vi "0 OCU.vi"(9 "Overview Image Ref In":T9, 10 "Map Name":T3="LPB Pool", 11 "Location of THINK":T13="127.0.0.1") -> ()   [LabVIEW 2011]
doc: "This is the current implementation of the operator control unit (OCU) for small RC boat controlled by a host computer. The following features are currently implemented:\n- override control of the rudden angle and sail value by control interface or using keys\n- ability to add missions before and during a run, by clicking and by using GPS location of the boat or an auxiliary GPS attached to the OCU computer\n- modification of tuning values used on the boat\n- indicators for all relevant system status information\n\nAuthors: Jared Kirschner, Jason Curtis"
uses:
  2-Think/2 Typedefs/setpoints to boat.ctl
  2-Think/2 Typedefs/sail setpt.ctl
  2-Think/2 Typedefs/rudder angle.ctl
  2-Think/2 Typedefs/Velocity.ctl
  2-Think/2 Typedefs/apparent wind direction.ctl
  2-Think/2 Typedefs/apparent wind speed.ctl
  2-Think/2 Typedefs/apparent wind.ctl
  2-Think/2 Typedefs/heading.ctl
  2-Think/2 Typedefs/UTM Location.ctl
  2-Think/2 Typedefs/Which Boat.ctl
  2-Think/2 Typedefs/generalized sensor status.ctl
  2-Think/2 Typedefs/indicator LED.ctl
  0x2-OCU-Think Comm/0x2 Typedefs/Current Waypoint.ctl
  2-Think/2 Typedefs/robot velocity.ctl
  0x2-OCU-Think Comm/0x2 Typedefs/manual override.ctl
  0 Typedefs/Location of Think.ctl
  0 Typedefs/Sail Position.ctl
  0 Typedefs/Rudder Position.ctl
  0 Typedefs/Apparent Wind Point of Sail.ctl
  0x2-OCU-Think Comm/0x2 Typedefs/ocuWaypoint.ctl
  0x2-OCU-Think Comm/0x2 Typedefs/Waypoints List.ctl
  2-Think/2 Classes/Waypoint/Waypoint.lvclass
  0 Typedefs/Mission Type Radio Buttons.ctl
  2-Think/2 Typedefs/rate of turn.ctl
  2-Think/2 Typedefs/pitch and roll.ctl
  2-Think/2 Typedefs/PI Constants.ctl
  2-Think/2 Typedefs/Goodness Weightings.ctl
  0 Typedefs/Maps.ctl
  <vilib>/vision/Image Controls.llb/IMAQ Image.ctl
  2-Think/2 Typedefs/Apparent Wind Mode.ctl
  2-Think/2 Classes/Missions/GenericMission/GenericMission.lvclass
  2-Think/2 Typedefs/UTM Circle.ctl
  0x2-OCU-Think Comm/0x2 Typedefs/RIO-OCU update controls.ctl
  2-Think/2 Typedefs/generalized actuator status.ctl
  2-Think/2 Typedefs/absolute wind direction.ctl
  2-Think/2 Typedefs/absolute wind speed.ctl
  2-Think/2 Typedefs/absolute water current vector.ctl
  2-Think/2 Typedefs/Goodness Fns Indicator.ctl
  2-Think/2 Typedefs/eStopCommand.ctl
  0x2-OCU-Think Comm/0x2 Typedefs/ocuMessage.ctl
  0x2-OCU-Think Comm/0x2 Typedefs/ocuCommands.ctl
  0x2-OCU-Think Comm/0x2 Typedefs/Control values.ctl
  0x2-OCU-Think Comm/0x2 Classes/NetworkStreams/Reader/readType.ctl
  2-Think/2 Globals/2 Global.vi
  0x2-OCU-Think Comm/0x2 Classes/NetworkStreams/Reader/NetworkStreamReader.lvclass
  0x2-OCU-Think Comm/0x2 Classes/NetworkStreams/Writer/NetworkStreamWriter.lvclass
  2-Think/2 Classes/Missions/RoundBuoy/RoundBuoy.lvclass
  2-Think/2 Classes/Missions/PassBuoys/PassBuoys.lvclass
  2-Think/2 Classes/Missions/StationKeeping/StationKeeping.lvclass
  2-Think/2 Classes/Missions/Drive/DriveTo.lvclass
panel:
  in  "Enable \nLocal GPS":bool
  out "Sensor Status":T1
  in  "GPS COM port":refnum<visa-resource-name>="COM1"
  in  "Additional inputs":T4(tab)
  in  "Manual Mission Input":enum32{"Drive", "Round", "Pass", "Station"}(tab)
  in  "Waypoint Location":enum32{"0", "1", "2", "3", "4"}(radio)
  in  "Buoy Side":enum32{"Starboard", "Port"}(radio)
  in  "Buoy to Round":enum32{"0", "1", "2", "3", "4"}(radio)
  in  "Starboard Buoy":enum32{"0", "1", "2", "3", "4"}(radio)=enum."1"
  in  "Port Buoy":enum32{"0", "1", "2", "3", "4"}(radio)
  in  "Buoy B":enum32{"0", "1", "2", "3", "4"}(radio)=enum."1"
  in  "Buoy A":enum32{"0", "1", "2", "3", "4"}(radio)
  in  "Add Mission":bool
  in  "Stored Locations Array":T5[](array[typedef])=[{"UTM Zone"=0.0, "Hemisphere"=enum."North", "East"=0.0, "North"=0.0}, {"UTM Zone"=0.0, "Hemisphere"=enum."North", "East"=0.0, "North"=0.0}, {"UTM Zone"=0.0, "Hemisphere"=enum."North", "East"=0.0, "North"=0.0}, {"UTM Zone"=0.0, "Hemisphere"=enum."North", "East"=0.0, "North"=0.0}, {"UTM Zone"=0.0, "Hemisphere"=enum."North", "East"=0.0, "North"=0.0}] {"North" format="%#_10f"; "East" format="%#_8f"}
  in  "Boat to Point 0":bool
  in  "Boat to Point 1":bool
  in  "Boat to Point 2":bool
  in  "Boat to Point 3":bool
  in  "Boat to Point 4":bool
  in  "Local to Point 4":bool
  in  "Local to Point 3":bool
  in  "Local to Point 2":bool
  in  "Local to Point 1":bool
  in  "Local to Point 0":bool
  in  "PI Constants":T6={"Proportional Gain"=1.0, "Integral Time"=0.0, "Derivative Time"=0.0}
  in  "Goodness Weightings":T7={"Target Importance"=0.98, "No Sail Importance"=1.0, "Change Importance"=0.05, "Pure Waypoint \nImportance"=0.0, "Pure Wind \nImportance"=0.0} {"Pure Wind \nImportance" min=0.0 step=0.2; "Pure Waypoint \nImportance" min=0.0 step=0.2; "Change Importance" min=0.0 step=0.2; "No Sail Importance" min=0.0 step=0.2; "Target Importance" min=0.0 step=0.2}
  in  "Update Constants":bool
  in  "No Sail Zone\nTuning Quotient":dbl=0.05 step=0.1
  in  "Heading Change\nWind Adjustment":dbl=0.2 step=0.1
  in  "Waypoint\nTuning Quotient":dbl=80.0 step=0.1
  in  "Apparent Wind Mode":T8 {"Desired Apparent\nWind Direction" step=0.1}
  in  "Runprotection Enabled":bool=TRUE
  in  "Let Sail Out on Windcross":bool
  in  "Shift Goal for currents":bool
  in  "Round Buoy Safety":dbl
  out "Battery Voltage":dbl
  out "Which Boat Am I?":T10
  out "Rudder Position":T11 scale=50.0..-50.0 scale format="%#.2g"
  out "Sail Position":T12
  out "Connected?":bool caption="Connection Status"
  in  "OVERRIDE SAIL?":bool
  in  "OVERRIDE RUDDER?":bool
  in  "Stop":bool
  in  "OCU Tab Control":enum32{"Mission [M]ap", "Detailed [T]elemetry"}(tab)
  in  "Map Mode":enum32{"M[i]ssion Edit", "M[o]nitoring"}(tab)
  in  "Load MDF":bool
  in  "Time(s)":dbl=300.0
  in  "Tolerance":dbl=3.0
  in  "Mission Entry Type":T14
  in  "Mission Def Filepath":path caption="MDF (Mission Definition File) path \n(leave blank for nothing)"
  in  "Reset Missions/Waypts":bool
  in  "Save Waypoints\nand PoI":bool
  out "# of Waypts":i32
  out "Robot Heading":T15 format="%05.1f"
  in  "Plot Colors":T16={"Target"=3381759, "No Sail"=16711680, "Change"=16756736, "Pure Waypt"=35080, "Pure Wind"=16860, "Combined"=16777228}
  out "Goodness Functions":picture
  out "Apparent Wind Direction\nPoint of Sail":T17 scale=0.0..360.0 scale format="%4d"
  out "Runprotection":bool
  in  "Log message":string caption="Log message (type and press enter)"
  in  "Save Image":bool
  out "Mission Map":T9(plugin-control)
  in  "Globals":T18(tab)
  out "Don't Tip?":bool
  out "Wind Sensor Status":T1
  out "Estimated Error":dbl
  out "Robot Heading":T15 format="%05.1f"
  out "Robot UTM Location":T5 {"North" format="%#_10f"; "East" format="%#_8f"}
  out "Robot Velocity":T19
  out "Robot\nRate of Turn":T20 format="%05.1f"
  out "Robot Pitch/Roll":T21 {"Roll" format="%05.1f"; "Pitch" format="%05.1f"}
  out "Absolute Wind":T22 {"East" format="%#_5g"}
  out "Apparent Wind Direction":T23
  out "Apparent Wind Speed":T24
  out "Apparent Wind":T25
  out "Crossing Wind":bool
  out "Setpoints to boat":T26
  out "Sail Position":T27
  out "Rudder Angle":T28
  out "Current Waypoint":T29
  in  "Reset to start":bool
  out "Manual Override":T30
  out "Waypoints Array":T31[](array[typedef]) {"UTM Location"."North" format="%#_10f"; "UTM Location"."East" format="%#_8f"}
  out "Waypoints Object Array":T32
  out "Mission Object Array":refnum<class "GenericMission.lvclass">[](array[class])
  out "Global No Sail Circles":T33[](array[typedef])
  # "Override\nSail: SHIFT"
  # "Override \nRudder: [W]"
  # "Full Out=RIGHT"
  # "Out=UP"
  # "In=DOWN"
  # "Full In=LEFT"
  # "PORT"
  # "STARB"
  # "[A]"
  # "[G]"
  # "Local GPS"
  # "<--[S]"
  # "[D]"
  # "[F]-->"
  # "Note: if THINK\nis on this computer,\nturning on local GPS will do strange things."
  # "HOWTO:\n1. save one or more points by moving GPS sensor to point, and pressing buttons below\n2. choose type of mission from tab control\n3. choose saved point(s) to load into mission. other params come from mission map input above\n4. click \"Add Mission\""
  # "P"
  # "S"
  # "O"
  # "O"
  # "A"
  # "B"
  # "HOWTO:\nchange values here, \nthen hit:"
  # "inputting missions:\nGo To Waypoint: set tolerance, and click on map.\nRound Buoy Port/Starboard: set tolerance, click.\nPass Between Buoys: Click one buoy location\nand drag to the other.\nStation Keeping: click southwest corner, drag to \nsoutheast corner. A square will be generated.\nTime(s) currently unimplemented.\nGlobal No-Sail Zone: click center of zone, drag to edge of\nzone. A circle with appropriate radius will be created."
  # "As Measured"
  # "Path Planning"
  # "From Planning Functions"
  # "(this is not a cluster because subitems\nare generated in parallel code)"
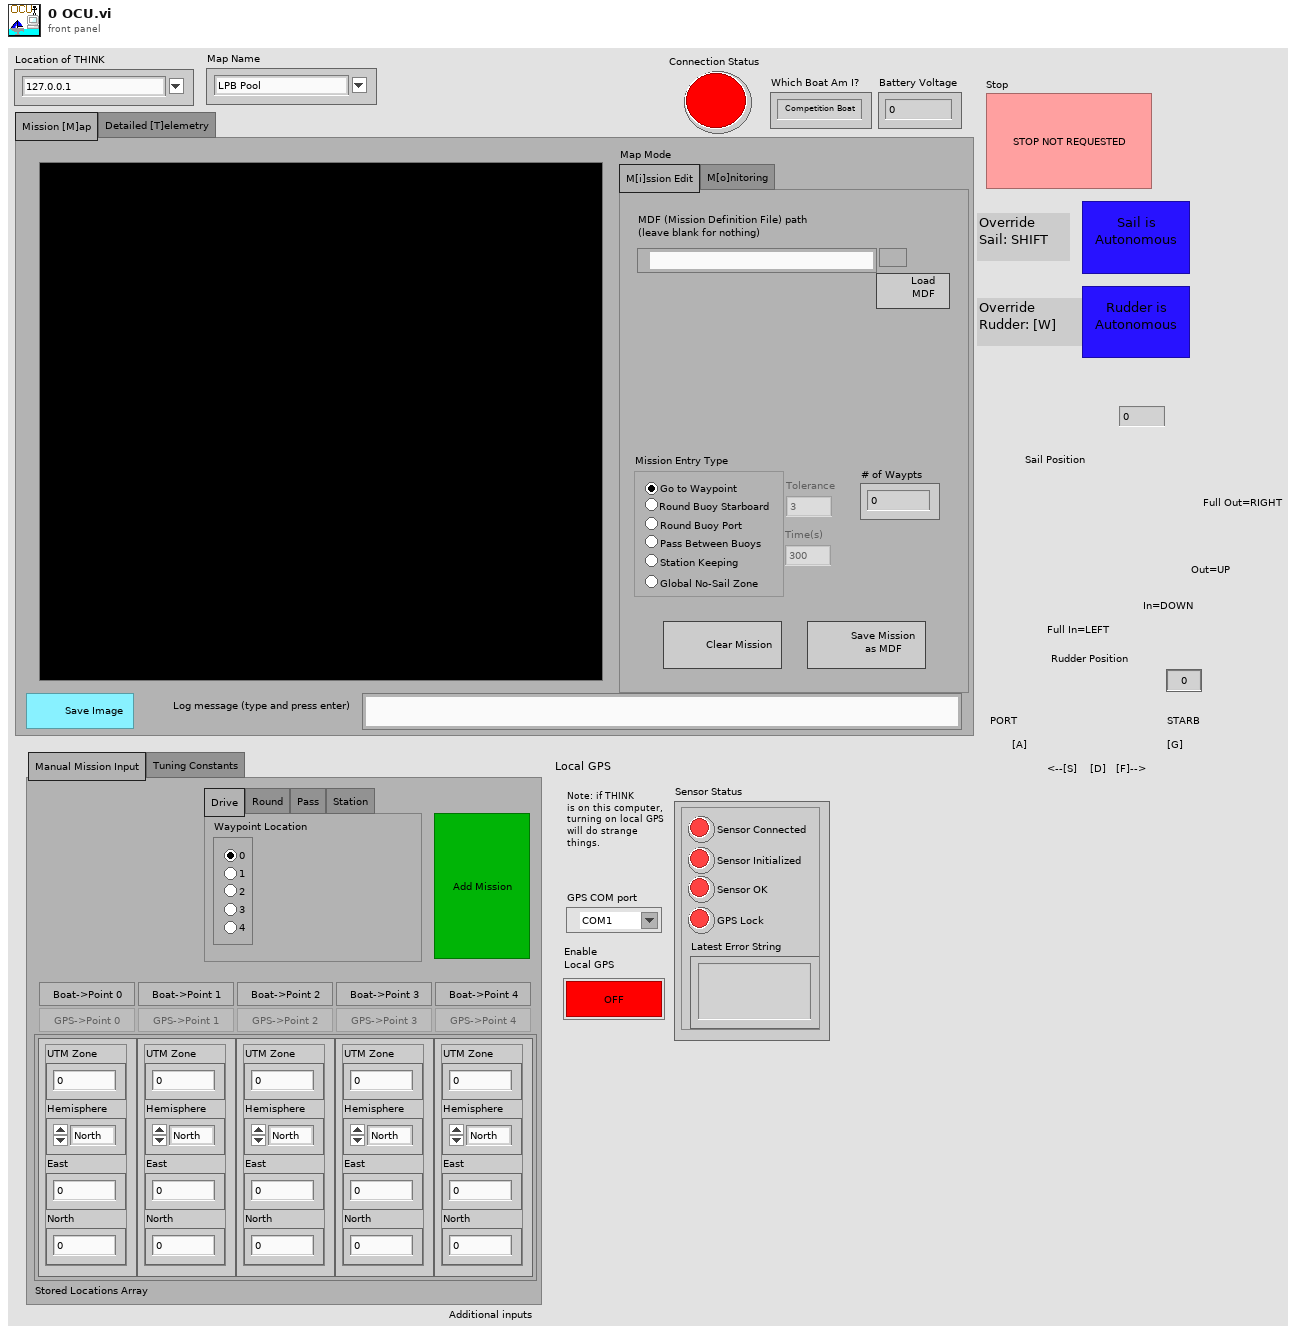
[diagram p1: front panel]
types:
  T1 = typedef "generalized sensor status.ctl" = cluster{"Sensor Connected":T2, "Sensor Initialized":T2, "Sensor OK":T2, "Latest Error String":string, "GPS Lock":T2}
  T2 = typedef "indicator LED.ctl" = bool
  T3 = typedef "Maps.ctl" = string
  T4 = enum32{"Manual Mission Input", "Tuning Constants"}
  T5 = typedef "UTM Location.ctl" = cluster{"UTM Zone":dbl, "Hemisphere":enum16{"North", "South"}, "East":dbl, "North":dbl}
  T6 = typedef "PI Constants.ctl" = cluster{"Proportional Gain":dbl, "Integral Time":dbl, "Derivative Time":dbl}
  T7 = typedef "Goodness Weightings.ctl" = cluster{"Target Importance":dbl, "No Sail Importance":dbl, "Change Importance":dbl, "Pure Waypoint \nImportance":dbl, "Pure Wind \nImportance":dbl}
  T8 = typedef "Apparent Wind Mode.ctl" = cluster{"Desired Apparent\nWind Direction":dbl, "On":bool}
  T9 = typedef "IMAQ Image.ctl" = refnum<image>
  T10 = typedef "Which Boat.ctl" = enum16{"Competition Boat", "Small RC", "Simulation"}
  T11 = typedef "Rudder Position.ctl" = dbl
  T12 = typedef "Sail Position.ctl" = dbl
  T13 = typedef "Location of Think.ctl" = string
  T14 = typedef "Mission Type Radio Buttons.ctl" = enum32{"Go to Waypoint", "Round Buoy Starboard", "Round Buoy Port", "Pass Between Buoys", "Station Keeping", "Global No-Sail Zone"}
  T15 = typedef "heading.ctl" = dbl
  T16 = cluster{"Target":u32, "No Sail":u32, "Change":u32, "Pure Waypt":u32, "Pure Wind":u32, "Combined":u32}
  T17 = typedef "Apparent Wind Point of Sail.ctl" = dbl
  T18 = enum32{"How Am I", "Where Am I", "What's Around Me", "Path Planning"}
  T19 = typedef "robot velocity.ctl" = cluster{"East":dbl, "North":dbl}
  T20 = typedef "rate of turn.ctl" = dbl
  T21 = typedef "pitch and roll.ctl" = cluster{"Pitch":dbl, "Roll":dbl}
  T22 = typedef "Velocity.ctl" = cluster{"East":dbl, "North":dbl}
  T23 = typedef "apparent wind direction.ctl" = dbl
  T24 = typedef "apparent wind speed.ctl" = dbl
  T25 = typedef "apparent wind.ctl" = cluster{"Toward Fore":dbl, "Toward Starboard":dbl}
  T26 = typedef "setpoints to boat.ctl" = cluster{"Sail Position":T27, "Rudder Angle":T28}
  T27 = typedef "sail setpt.ctl" = dbl
  T28 = typedef "rudder angle.ctl" = dbl
  T29 = typedef "Current Waypoint.ctl" = i32
  T30 = typedef "manual override.ctl" = cluster{"Override Active Rudder":bool, "Setpoints":T26, "Override Active Sail":bool}
  T31 = typedef "ocuWaypoint.ctl" = cluster{"Tolerance (m)":dbl, "UTM Location":T5}
  T32 = typedef "Waypoints List.ctl" = refnum<class "Waypoint.lvclass">[]
  T33 = typedef "UTM Circle.ctl" = cluster{"UTM Zone":dbl, "Hemisphere":enum16{"North", "South"}, "East":dbl, "North":dbl, "Radius":dbl}
  T34 = typedef "RIO-OCU update controls.ctl" = cluster{"Sensor Status":T1, "Battery Voltage":dbl, "Rudder Actuator Status":T35, "Sail Actuator Status":T35, "Which Boat Am I?":T10, "Robot Velocity":T19, "Robot UTM Location":T5, "Robot\nHeading ":T15, "Robot\nRate of Turn":T20, "Robot Pitch/Roll":T21, "Apparent Wind":T25, "Apparent Wind\nSpeed":T24, "Apparent Wind\nDirection (º)":T23, "Absolute Wind":T22, "Absolute Wind\nDirection (º)":T36, "Absolute Wind\nSpeed":T37, "Absolute Water Current Vector":T38, "Rudder Angle":T28, "Sail Position":T27, "Manual Override Cluster":T30, "Setpoints to boat":T26, "Current Waypoint":T29, "Think freq.":dbl, "Sense freq.":dbl, "Act freq.":dbl, "E-stop freq.":dbl, "Network \nfreq.":dbl, "Network \nLoop Iterations":i64, "E-Stop":bool, "Serialized Waypoint Array":string, "Serialized Mission Queue Elements":string, "Goodness Functions":T39, "Global No Sail Circles":T33[], "Runprotection":bool, "Optimal Heading":dbl, "Crossing Wind":bool, "Estimated Error":dbl, "Don't Tip?":bool}
  T35 = typedef "generalized actuator status.ctl" = cluster{"Actuator Connected":T2}
  T36 = typedef "absolute wind direction.ctl" = dbl
  T37 = typedef "absolute wind speed.ctl" = dbl
  T38 = typedef "absolute water current vector.ctl" = cluster{"Direction":T23, "Magnitude":T23}
  T39 = typedef "Goodness Fns Indicator.ctl" = cluster{dbl, dbl, dbl[][]}
  T40 = typedef "0-Image Descriptor.ctl" = cluster{"Upper-Left Corner Coordinates":T5, "Meters/Pixel":dbl}
  T41 = typedef "eStopCommand.ctl" = enum16{"Reset E-Stop", "Get E-Stop", "Set E-Stop"}
  T42 = typedef "NetworkStreamReader.lvclass/readType.ctl" = enum16{"Next in buffer", "Most current"}
  T43 = cluster{"Image Ref Out":T9, "Image Descriptor":T40}
  T44 = typedef "ocuMessage.ctl" = cluster{"OCU Command":T45, "Data":variant}
  T45 = typedef "ocuCommands.ctl" = enum16{"Pass", "Send override", "Add waypoint", "Set waypoint number", "Stop", "Add Mission", "Reset Missions/Waypts", "Edit Control Values", "Add Global No-Sail", "Log Message"}
  T46 = typedef "Control values.ctl" = cluster{"Goodness Weightings":T7, "PI Constants":T6, "No Sail Zone\nTuning Quotient":dbl, "Heading Change Wind Adjustment":dbl, "Waypoint Tuning Quotient":dbl, "Apparent Wind Mode":T8, "RP Autonomous":bool, "Let Sail Out on Windcross":bool, "Shift Goal for currents":bool, "Round Buoy Safety":dbl}
  T47 = enum8{"Enabled", "Disabled", "Disabled and Grayed Out"}
  T48 = typedef "eventvkey.ctl" = enum16{"ASCII", "Enter", "Return", "Shift", "Ctrl", "Alt", "Cmd", "Opt", "Caps", "NumLock", "Clear", "Break", "Up", "Down", "Left", "Right", "Insert", "Delete", "Home", "End", "PageUp", "PageDown", "Escape", "Help", "Pause", "ScrollLock", "F1", "F2", "F3", "F4", "F5", "F6", "F7", "F8", "F9", "F10", "F11", "F12", "F13", "F14", "F15", "F16", "F17", "F18", "F19", "F20", "F21", "F22", "F23", "F24", "Play", "VolumeUp", "VolumeDown", "Mute", "Two Byte Char"}
  T49 = cluster{"Global Rectangle":i32[], "Contours":cluster{"Contour Type":u32, "ROI Type":u32, "Points":i32[]}[]}
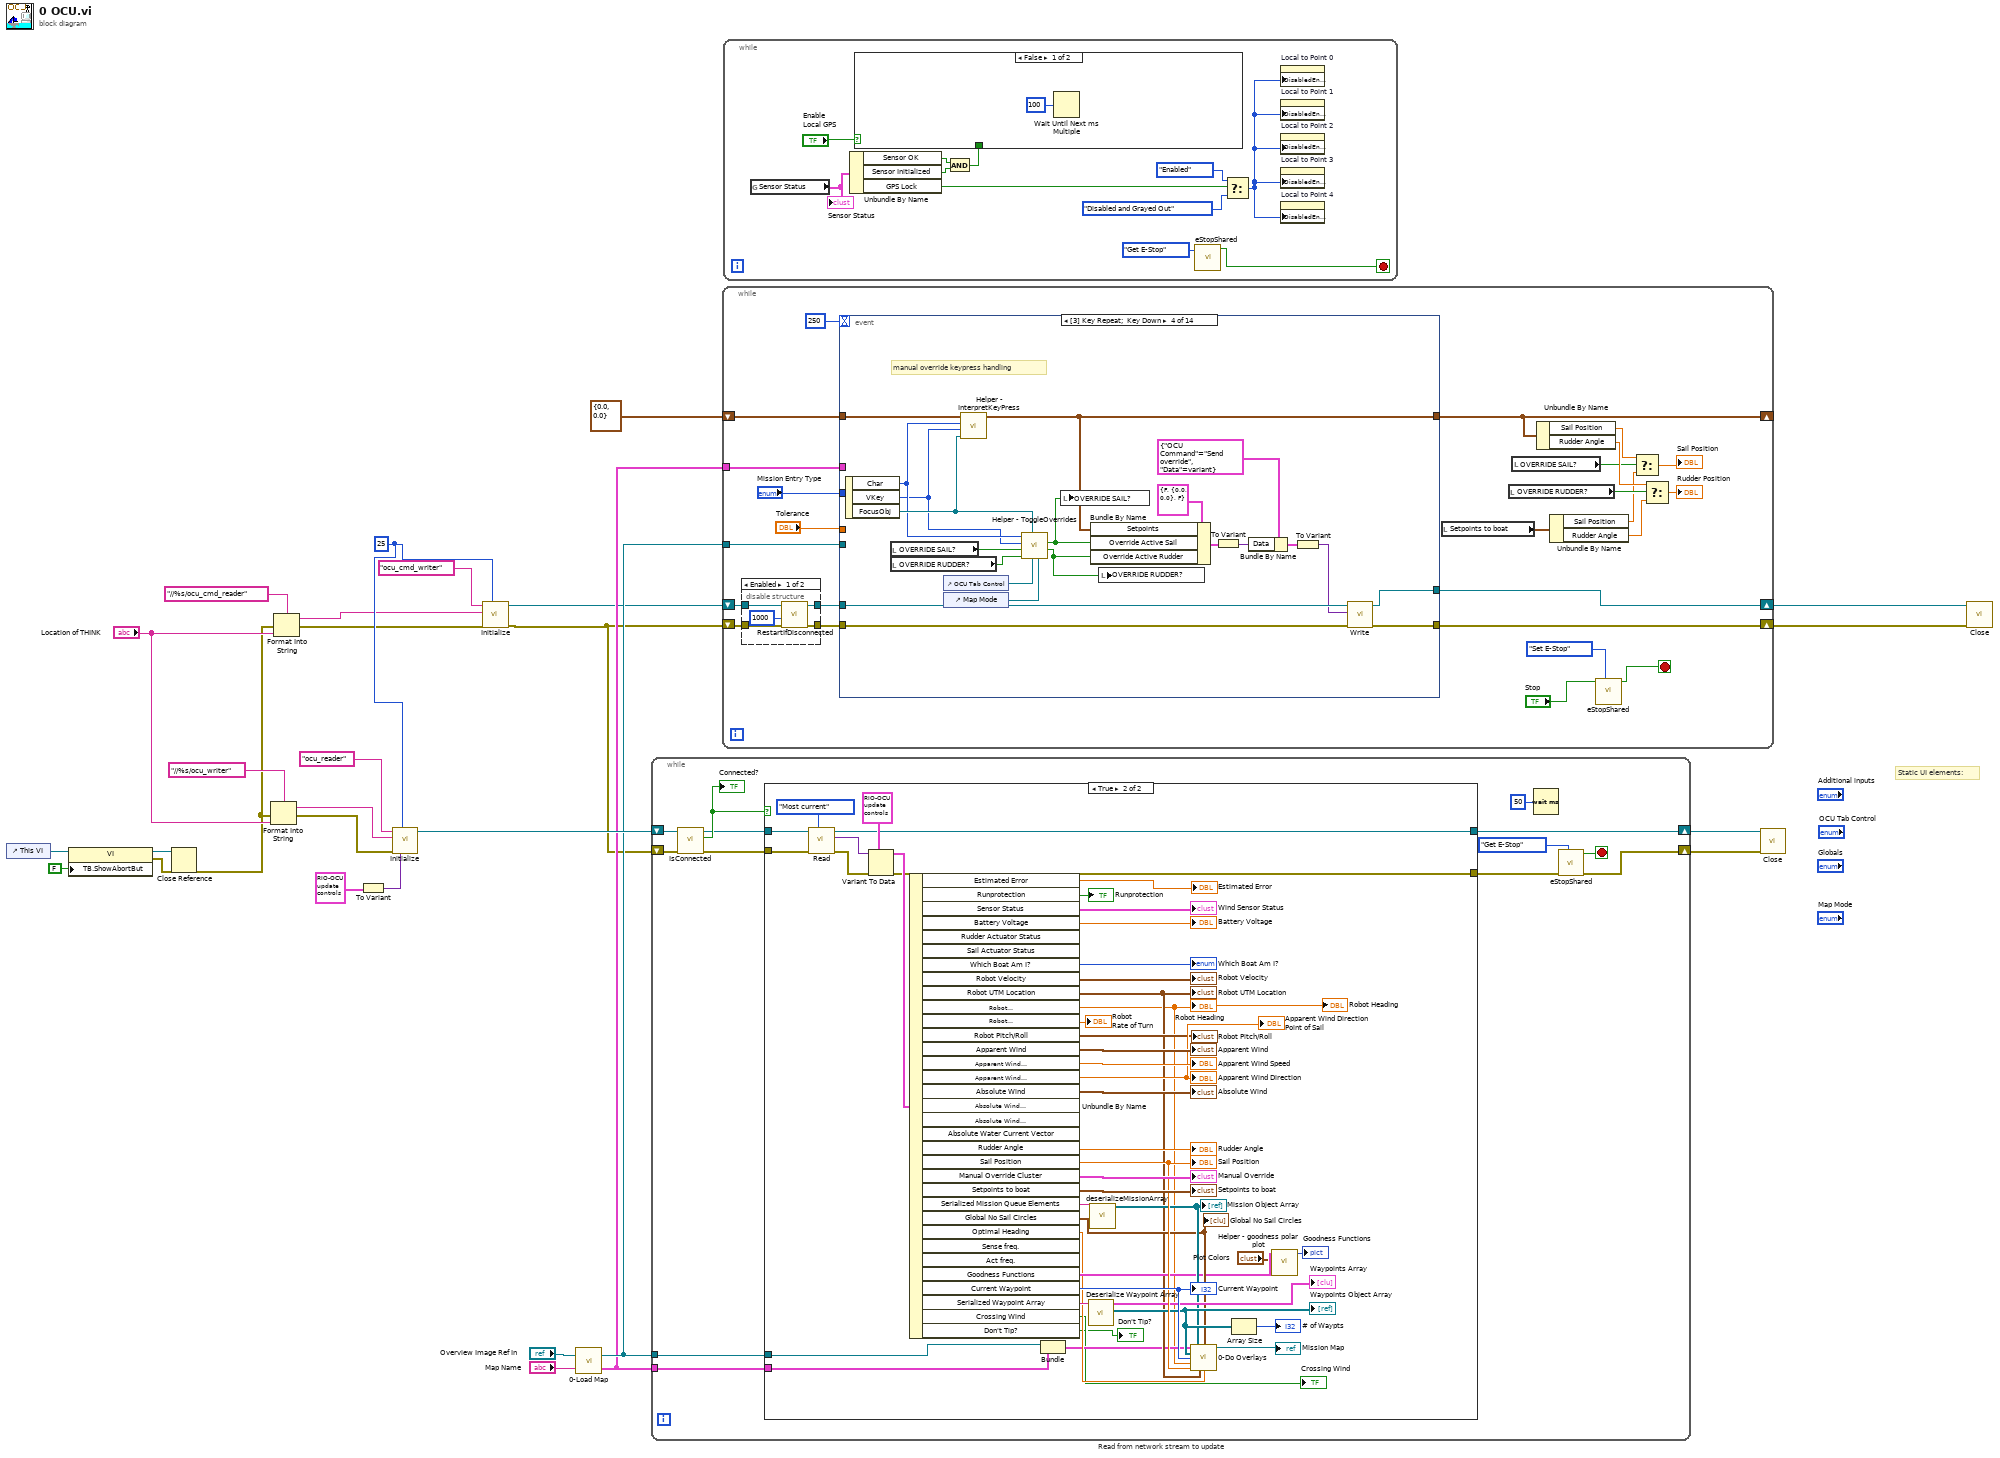
[diagram p0: block diagram]
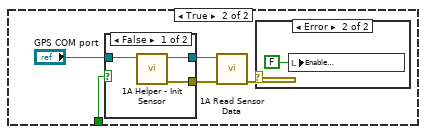
[diagram p2: hidden frame]
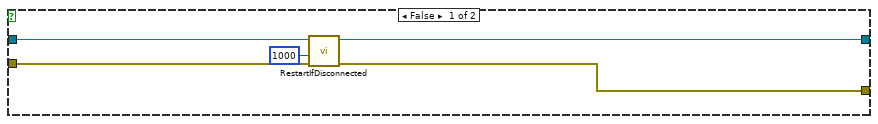
[diagram p5: hidden frame]
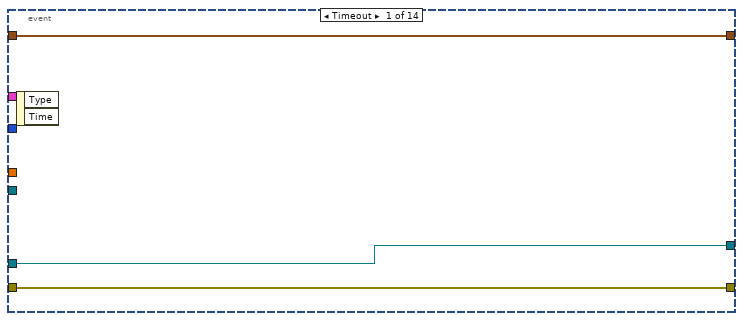
[diagram p7: hidden frame]
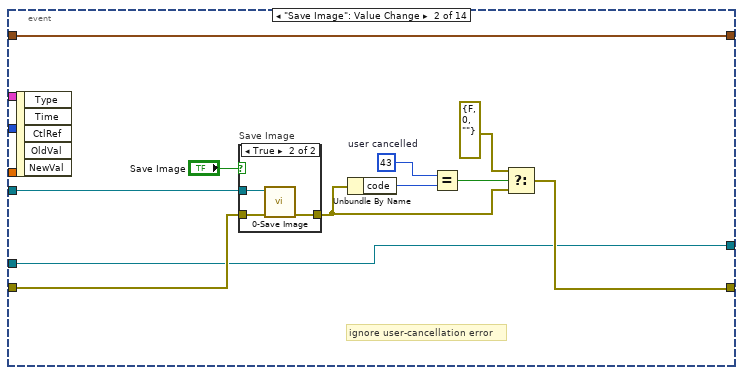
[diagram p8: hidden frame]
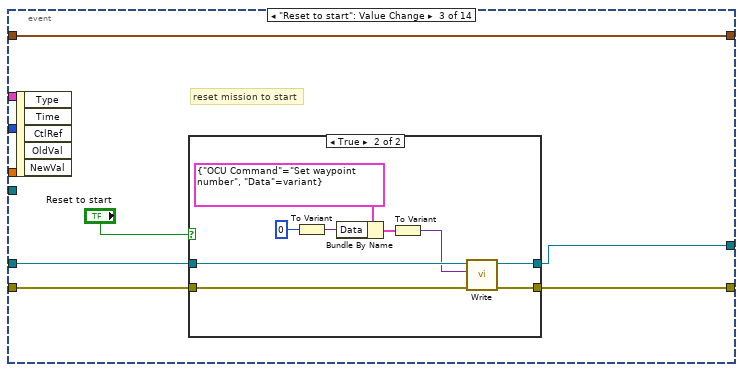
[diagram p10: hidden frame]
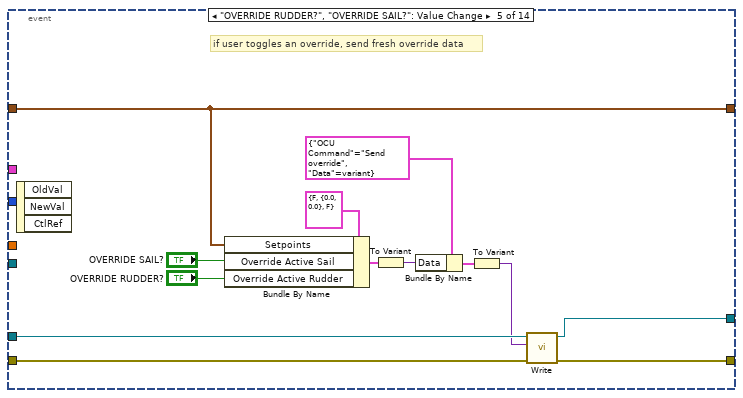
[diagram p12: hidden frame]
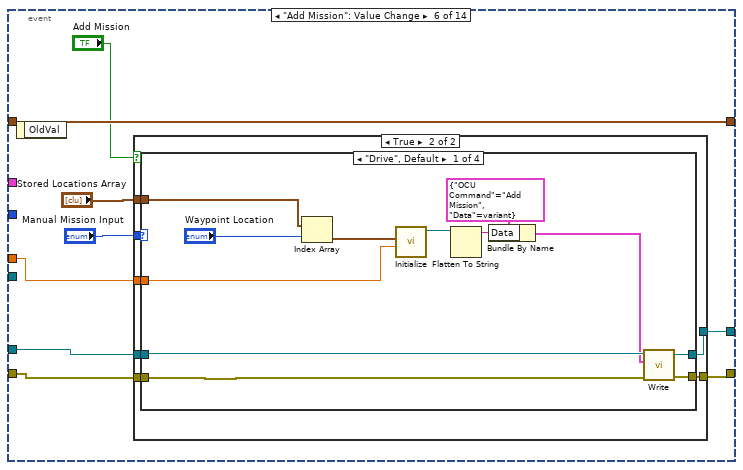
[diagram p13: hidden frame]
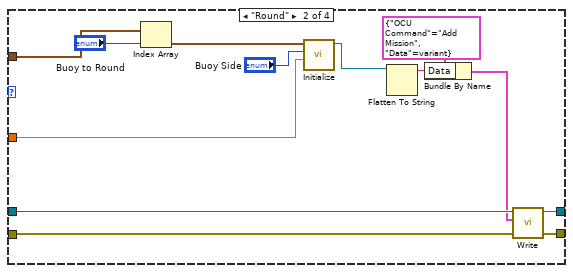
[diagram p15: hidden frame]
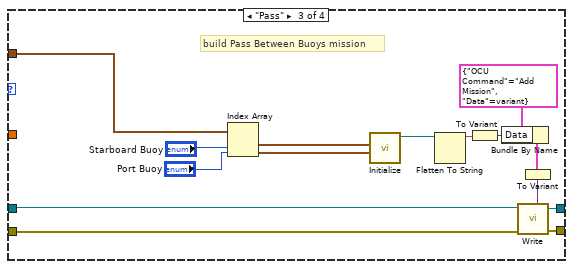
[diagram p16: hidden frame]
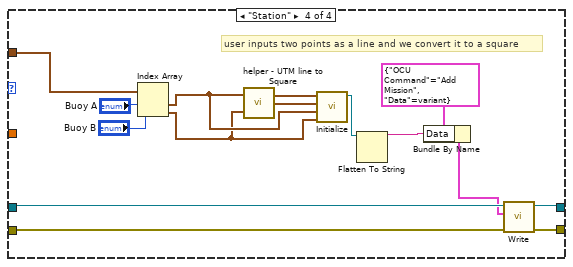
[diagram p17: hidden frame]
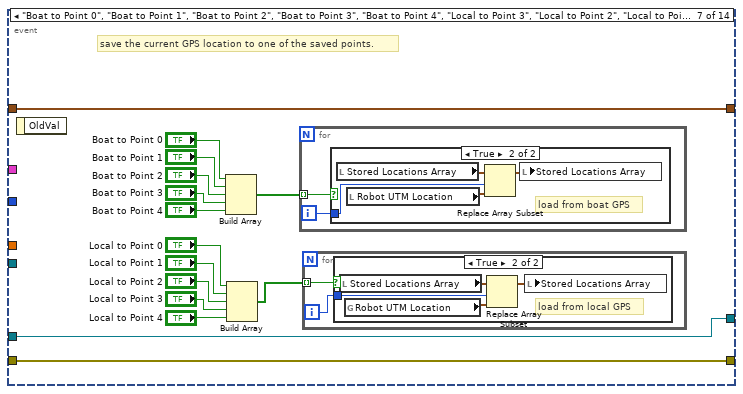
[diagram p18: hidden frame]
diagram:
  w27 = 25 ("writer buffer size")
  # "Static UI elements:"
  n1 = control-ref of="This VI"() -> (w17:refnum<vi>)
  n2 = property class="VI"(reference=w17, "TB.ShowAbortBut"=FALSE ("Tool Bar:Show Abort Button")) -> (reference out=w15:refnum<vi>, error out=w14:errorcluster)  [unwired: 1 in]
  n3 = Close Reference(reference=w15, error in (no error)=w14) -> (error out=w13:errorcluster)
  n4 = Format Into String(format string="//%s/ocu_writer", error in=w13, "Location of THINK") -> (resulting string=w7:string, error out=w11:errorcluster)  [unwired: 1 in]
  n5 = Format Into String(format string="//%s/ocu_cmd_reader", error in=w13, "Location of THINK") -> (resulting string=w5:string, error out=w12:errorcluster)  [unwired: 1 in]
  n6 = To Variant(anything=T34 {"Sensor Status"={"Sensor Connected"=FALSE, "Sensor Initialized"=FALSE, "Sensor OK"=FALSE, "Latest Error String"="", "GPS Lock"=FALSE}, "Battery Voltage"=0.0, "Rudder Actuator Status"={"Actuator Connected"=FALSE}, "Sail Actuator Status"={"Actuator Connected"=FALSE}, "Which Boat Am I?"=enum."Competition Boat", "Robot Velocity"={"East"=0.0, "North"=0.0}, "Robot UTM Location"={"UTM Zone"=0.0, "Hemisphere"=enum."North", "East"=0.0, "North"=0.0}, "Robot\nHeading "=0.0, "Robot\nRate of Turn"=0.0, "Robot Pitch/Roll"={"Pitch"=0.0, "Roll"=0.0}, "Apparent Wind"={"Toward Fore"=0.0, "Toward Starboard"=0.0}, "Apparent Wind\nSpeed"=0.0, "Apparent Wind\nDirection (º)"=0.0, "Absolute Wind"={"East"=0.0, "North"=0.0}, "Absolute Wind\nDirection (º)"=0.0, "Absolute Wind\nSpeed"=0.0, "Absolute Water Current Vector"={"Direction"=0.0, "Magnitude"=0.0}, "Rudder Angle"=0.0, "Sail Position"=0.0, "Manual Override Cluster"={"Override Active Rudder"=FALSE, "Setpoints"={"Sail Position"=0.0, "Rudder Angle"=0.0}, "Override Active Sail"=FALSE}, "Setpoints to boat"={"Sail Position"=0.0, "Rudder Angle"=0.0}, "Current Waypoint"=0, "Think freq."=0.0, "Sense freq."=0.0, "Act freq."=0.0, "E-stop freq."=0.0, "Network \nfreq."=0.0, "Network \nLoop Iterations"=0, "E-Stop"=FALSE, "Serialized Waypoint Array"="", "Serialized Mission Queue Elements"="", "Goodness Functions"={0.0, 0.0, []}, "Global No Sail Circles"=[], "Runprotection"=FALSE, "Optimal Heading"=0.0, "Crossing Wind"=FALSE, "Estimated Error"=0.0, "Don't Tip?"=FALSE} ("RIO->OCU update data")) -> (Variant=w26:variant)
  n7 = call "Initialize.vi"("Default return"=w26, "reader buffer size"=w27, "error in (no error)"=w11, "writer url"=w7, "reader name"="ocu_reader" ("writer name")) -> ("NetworkStreamWriter out"=w28:refnum<class "NetworkStreamReader.lvclass">)  [unwired: 4 in, 2 out]
  n8 = call "Initialize.vi"("writer buffer size"=w27, "error in (no error)"=w12, "reader url"=w5, "writer name"="ocu_cmd_writer") -> ("error out"=w1:errorcluster, "NetworkStreamWriter out"=w2:refnum<class "NetworkStreamWriter.lvclass">)  [unwired: 5 in, 1 out]
  n9 = call "0-Load Map.vi"("Map Name"="Map Name", "Image Ref In"="Overview Image Ref In") -> ("Image Descriptor"=w9:T40, "Image Ref Out"=w23:T9)
  n10 = while "Read from network stream to update" {
    shift-right: [w42] -> w25
    shift-left: w28 -> [w37]
    shift-right: [w35] -> w24
    shift-left: w1 -> [w36]
    tunnel: w23 -> [w39]
    tunnel: w9 -> [w38]
    stop <- w40 stop-if-true
    n11 = call "IsConnected.vi"("error in (no error)"=w36, "NetworkStreamReader in"=w37) -> ("error out"=w31:errorcluster, "Connected?"=w33:bool, "NetworkStreamReader out"=w32:refnum<class "NetworkStreamReader.lvclass">)  [unwired: 7 in]
    "Connected?" <- w33
    n12 = case shown="True" w33 {
      tunnel: [w45 w88] -> w42
      tunnel: w39 -> [_ w65]
      tunnel: w38 -> [_ w64]
      tunnel: w32 -> [w47 w72]
      tunnel: w31 -> [w46 w71]
      tunnel: [w44 w70] -> w30
      frame False {
        n13 = call "RestartIfDisconnected.vi"("error in (no error)"=w46, "connection timeout"=1000, "NetworkStreamReader in"=w47) -> ("error out"=w44:errorcluster, "NetworkStreamReader out"=w45:refnum<class "NetworkStreamReader.lvclass">)  [unwired: 7 in]
      }
      frame True {
        n14 = call "Read.vi"("Read Type"=readType."Most current", "error in (no error)"=w71, "NetworkStreamReader in"=w72) -> ("error out"=w91:errorcluster, "element"=w90:variant, "NetworkStreamReader out"=w88:refnum<class "NetworkStreamReader.lvclass">)  [unwired: 4 in, 2 out]
        n15 = Variant To Data(error in=w91, type=T34 {"Sensor Status"={"Sensor Connected"=FALSE, "Sensor Initialized"=FALSE, "Sensor OK"=FALSE, "Latest Error String"="", "GPS Lock"=FALSE}, "Battery Voltage"=0.0, "Rudder Actuator Status"={"Actuator Connected"=FALSE}, "Sail Actuator Status"={"Actuator Connected"=FALSE}, "Which Boat Am I?"=enum."Competition Boat", "Robot Velocity"={"East"=0.0, "North"=0.0}, "Robot UTM Location"={"UTM Zone"=0.0, "Hemisphere"=enum."North", "East"=0.0, "North"=0.0}, "Robot\nHeading "=0.0, "Robot\nRate of Turn"=0.0, "Robot Pitch/Roll"={"Pitch"=0.0, "Roll"=0.0}, "Apparent Wind"={"Toward Fore"=0.0, "Toward Starboard"=0.0}, "Apparent Wind\nSpeed"=0.0, "Apparent Wind\nDirection (º)"=0.0, "Absolute Wind"={"East"=0.0, "North"=0.0}, "Absolute Wind\nDirection (º)"=0.0, "Absolute Wind\nSpeed"=0.0, "Absolute Water Current Vector"={"Direction"=0.0, "Magnitude"=0.0}, "Rudder Angle"=0.0, "Sail Position"=0.0, "Manual Override Cluster"={"Override Active Rudder"=FALSE, "Setpoints"={"Sail Position"=0.0, "Rudder Angle"=0.0}, "Override Active Sail"=FALSE}, "Setpoints to boat"={"Sail Position"=0.0, "Rudder Angle"=0.0}, "Current Waypoint"=0, "Think freq."=0.0, "Sense freq."=0.0, "Act freq."=0.0, "E-stop freq."=0.0, "Network \nfreq."=0.0, "Network \nLoop Iterations"=0, "E-Stop"=FALSE, "Serialized Waypoint Array"="", "Serialized Mission Queue Elements"="", "Goodness Functions"={0.0, 0.0, []}, "Global No Sail Circles"=[], "Runprotection"=FALSE, "Optimal Heading"=0.0, "Crossing Wind"=FALSE, "Estimated Error"=0.0, "Don't Tip?"=FALSE} ("RIO->OCU update data"), Variant=w90) -> (data=w87:T34, error out=w70:errorcluster)
        n16 = Unbundle By Name(w87) -> ("Estimated Error"=→"Estimated Error":dbl, "Runprotection"=→"Runprotection":bool, "Sensor Status"=→"Wind Sensor Status":T1, "Battery Voltage"=→"Battery Voltage":dbl, "Which Boat Am I?"=→"Which Boat Am I?":T10, "Robot Velocity"=→"Robot Velocity":T19, "Robot UTM Location"=w54:T5, "Robot\nHeading"=w50:T15, "Robot\nRate of Turn"=→"Robot\nRate of Turn":T20, "Robot Pitch/Roll"=→"Robot Pitch/Roll":T21, "Apparent Wind"=→"Apparent Wind":T25, "Apparent Wind\nSpeed"=→"Apparent Wind Speed":T24, "Apparent Wind\nDirection (º)"=→"Apparent Wind Direction" →"Apparent Wind Direction\nPoint of Sail":T23, "Absolute Wind"=→"Absolute Wind":T22, "Rudder Angle"=→"Rudder Angle":T28, "Sail Position"=w73:T27, "Manual Override Cluster"=→"Manual Override":T30, "Setpoints to boat"=→"Setpoints to boat":T26, "Serialized Mission Queue Elements"=w63:string, "Global No Sail Circles"=w59:T33[], "Optimal Heading"=w53:dbl, "Goodness Functions"=w57:T39, "Current Waypoint"=w74:T29, "Serialized Waypoint Array"=w69:string, "Crossing Wind"=→"Crossing Wind":bool, "Don't Tip?"=→"Don't Tip?":bool)  [unwired: 7 out]
        "Robot UTM Location" <- w54
        "Robot Heading" <- w50
        "Sail Position" <- w73
        "Current Waypoint" <- w74
        "Global No Sail Circles" <- w59
        "Robot Heading" <- w50
        n17 = Bundle("Image Ref Out"=w65, "Image Descriptor"=w64) -> (w52:T43)  [unwired: 1 in]
        n18 = call "Deserialize Waypoint Array.vi"("Serialized Waypoint Array"=w69) -> ("Waypoints Object Array"=w67:T32, "Waypoints Array"=→"Waypoints Array":T31[])  [unwired: 9 in]
        "Waypoints Object Array" <- w67
        n19 = call "deserializeMissionArray.vi"("Serialized Mission Array"=w63) -> ("Mission Object Array"=w62:refnum<class "GenericMission.lvclass">[])  [unwired: 9 in, 1 out]
        "Mission Object Array" <- w62
        n20 = call "0-Do Overlays.vi"("Image Reference\nand Descriptor"=w52, "Missions"=w62, "No Sail Circles"=w59, "Waypoints"=w67, "Current Waypoint #"=w74, "Heading"=w50, "Sail Position"=w73, "Robot UTM Location"=w54, "Optimal Heading"=w53) -> ("Image out"=→"Mission Map":T9)  [unwired: 6 in]
        n21 = Array Size(array=w67) -> (size(s)=→"# of Waypts":i32)
        n22 = call "Helper - goodness polar plot.vi"("Plot Colors"="Plot Colors", "Goodness Fns In"=w57) -> ("Goodness Functions Polar Plot"=→"Goodness Functions":picture)  [unwired: 9 in]
      }
    }
    n23 = Wait (ms)(milliseconds to wait=u32 50 ("millisecond multiple")) -> ()  [unwired: 1 out]
    n24 = call "eStopShared.vi"("Command"=eStopCommand."Get E-Stop", "Error In"=w30) -> ("Error Out"=w35:errorcluster, "E-Stop Out"=w40:bool)  [unwired: 8 in]
  }
  n25 = while {
    shift-right: [w115] -> w18
    shift-left: w1 -> [w97]
    shift-right: [w109] -> _
    shift-left: T26 {"Sail Position"=0.0, "Rudder Angle"=0.0} ("Setpoints") -> [w117]
    shift-right: [w111] -> w19
    shift-left: w2 -> [w98]
    tunnel: w23 -> [w110]
    tunnel: w9 -> [w108]
    stop <- w114 stop-if-true
    n26 = disable-structure shown="Enabled" {
      disable-tunnel: w98 -> [w122 w124]
      disable-tunnel: w97 -> [w121 w123]
      disable-tunnel: [w120 w124] -> w93
      disable-tunnel: [w119 w123] -> w96
      frame Enabled {
        n27 = call "RestartIfDisconnected.vi"("error in (no error)"=w121, "connection timeout"=1000, "NetworkStreamWriter in"=w122) -> ("error out"=w119:errorcluster, "NetworkStreamWriter out"=w120:refnum<class "NetworkStreamWriter.lvclass">)  [unwired: 7 in]
      }
      frame Disabled {
      }
    }
    n28 = event shown="[3] Key Repeat;  Key Down" {
      selector: _ -> [_ _ _ _ _ _ _ _ _ _ _ _ _ _]
      dyn-events: _ -> [_ _ _ _ _ _ _ _ _ _ _ _ _ _]
      timeout: 250 -> [_ _ _ _ _ _ _ _ _ _ _ _ _ _]
      tunnel: w117 -> [w127 w134 w148 w180 w183 w200 w274 w298 w331 w347 w356 w397 w415 w535]
      tunnel: [w127 w134 w148 w178 w183 w200 w274 w298 w331 w347 w356 w397 w415 w535] -> w109
      tunnel: w96 -> [w125 w132 w145 w175 w190 w201 w272 w295 w323 w346 w354 w395 w414 w536]
      tunnel: [w125 w129 w143 w174 w189 w198 w272 w293 w321 w346 w353 w393 w412 w536] -> w115
      tunnel: w93 -> [w126 w128 w146 w177 w192 w202 w273 w296 w322 w345 w352 w396 w410 w537]
      tunnel: [w126 w128 w144 w176 w191 w197 w273 w294 w324 w345 w351 w394 w411 w537] -> w111
      tunnel: w110 -> [_ w133 _ _ _ _ _ _ _ _ _ _ _ _]
      tunnel: w108 -> [_ _ _ _ _ _ _ _ _ _ _ _ w413 _]
      tunnel: "Mission Entry Type" -> [_ _ _ _ _ _ _ _ _ _ _ _ w409 _]
      tunnel: "Tolerance" -> [_ _ _ _ _ w199 _ _ _ _ _ _ w408 _]
      event Timeout {
        n29 = event-data() -> ()  [unwired: 1 in, 2 out]
      }
      event "Save Image": Value Change {
        w137 = 43  # user cancelled
        # "ignore user-cancellation error"
        n30 = event-data() -> ()  [unwired: 1 in, 5 out]
        n31 = case "Save Image" shown="True" "Save Image" {
          tunnel: w132 -> [w139 w142]
          tunnel: [w139 w141] -> w131
          tunnel: w133 -> [_ w140]
          frame False {
          }
          frame True {
            n32 = call "0-Save Image.vi"("Error In"=w142, "Image in"=w140) -> ("Error Out"=w141:errorcluster)  [unwired: 9 in]
          }
        }
        n33 = Unbundle By Name(w131) -> ("code"=w138:i32)
        n34 = Equal?(x=w137, y=w138) -> (x = y?=w136:bool)
        n35 = Select(t=errorcluster {"status"=FALSE, "code"=0, "source"=""}, s=w136, f=w131) -> (s? t:f=w129:errorcluster)
      }
      event "Reset to start": Value Change {
        # "reset mission to start"
        n36 = event-data() -> ()  [unwired: 1 in, 5 out]
        n37 = case shown="True" "Reset to start" {
          tunnel: w146 -> [w150 w156]
          tunnel: w145 -> [w149 w157]
          tunnel: [w150 w159] -> w144
          tunnel: [w149 w158] -> w143
          frame False {
          }
          frame True {
            n38 = To Variant(anything=T29 0 ("Current Waypoint")) -> (Variant=w154:variant)
            n39 = Bundle By Name(cluster=T44 {"OCU Command"=enum."Set waypoint number", "Data"=variant}, "Data"=w154) -> (w152:T44)
            n40 = To Variant(anything=w152) -> (Variant=w151:variant)
            n41 = call "Write.vi"("error in (no error)"=w157, "element"=w151, "NetworkStreamWriter in"=w156) -> ("error out"=w158:errorcluster, "NetworkStreamWriter out"=w159:refnum<class "NetworkStreamWriter.lvclass">)  [unwired: 6 in, 1 out]
          }
        }
      }
      event Key Repeat; Key Down {
        # "manual override keypress handling"
        n42 = event-data() -> ("Char"=w167:i16, "VKey"=w166:T48, "FocusObj"=w168:refnum<vi>)  [unwired: 1 in]
        n43 = local read "OVERRIDE SAIL?"() -> (w165:bool)
        n44 = local read "OVERRIDE RUDDER?"() -> (w164:bool)
        n45 = control-ref of="OCU Tab Control"() -> (w161:refnum<vi>)
        n46 = control-ref of="Map Mode"() -> (w160:refnum<vi>)
        n47 = call "Helper - InterpretKeyPress.vi"("FocusObj"=w168, "VKey"=w166, "Char"=w167, "Command In"=w180) -> ("Command Out"=w178:T26)  [unwired: 7 in]
        n48 = call "Helper - ToggleOverrides.vi"("Map Mode Tab Control Ref"=w160, "OCU Tab Control Ref"=w161, "FocusObj"=w168, "Rudder Override?"=w164, "Sail Override?"=w165, "VKey"=w166, "Char"=w167) -> ("Override Rudder"=w163:bool, "Override Sail"=w162:bool)  [unwired: 3 in]
        n49 = local write "OVERRIDE SAIL?"(w162) -> ()
        n50 = Bundle By Name(cluster=T30 {"Override Active Rudder"=FALSE, "Setpoints"={"Sail Position"=0.0, "Rudder Angle"=0.0}, "Override Active Sail"=FALSE} ("Manual Override Cluster"), "Setpoints"=w178, "Override Active Sail"=w162, "Override Active Rudder"=w163) -> (w170:T30)
        n51 = local write "OVERRIDE RUDDER?"(w163) -> ()
        n52 = To Variant(anything=w170) -> (Variant=w173:variant)
        n53 = Bundle By Name(cluster=T44 {"OCU Command"=enum."Send override", "Data"=variant}, "Data"=w173) -> (w172:T44)
        n54 = To Variant(anything=w172) -> (Variant=w169:variant)
        n55 = call "Write.vi"("error in (no error)"=w175, "element"=w169, "NetworkStreamWriter in"=w177) -> ("error out"=w174:errorcluster, "NetworkStreamWriter out"=w176:refnum<class "NetworkStreamWriter.lvclass">)  [unwired: 6 in, 1 out]
      }
      event "OVERRIDE RUDDER?", "OVERRIDE SAIL?": Value Change {
        # "if user toggles an override, send fresh override data"
        n56 = event-data() -> ()  [unwired: 1 in, 3 out]
        n57 = Bundle By Name(cluster=T30 {"Override Active Rudder"=FALSE, "Setpoints"={"Sail Position"=0.0, "Rudder Angle"=0.0}, "Override Active Sail"=FALSE} ("Manual Override Cluster"), "Setpoints"=w183, "Override Active Sail"="OVERRIDE SAIL?", "Override Active Rudder"="OVERRIDE RUDDER?") -> (w185:T30)
        n58 = To Variant(anything=w185) -> (Variant=w188:variant)
        n59 = Bundle By Name(cluster=T44 {"OCU Command"=enum."Send override", "Data"=variant}, "Data"=w188) -> (w187:T44)
        n60 = To Variant(anything=w187) -> (Variant=w184:variant)
        n61 = call "Write.vi"("error in (no error)"=w190, "element"=w184, "NetworkStreamWriter in"=w192) -> ("error out"=w189:errorcluster, "NetworkStreamWriter out"=w191:refnum<class "NetworkStreamWriter.lvclass">)  [unwired: 6 in, 1 out]
      }
      event "Add Mission": Value Change {
        n62 = event-data() -> ()  [unwired: 1 in, 1 out]
        n63 = case shown="True" "Add Mission" {
          tunnel: w202 -> [w204 w211]
          tunnel: w201 -> [w203 w210]
          tunnel: w199 -> [_ w209]
          tunnel: [w203 w208] -> w198
          tunnel: [w204 w207] -> w197
          tunnel: "Manual Mission Input" -> [_ w206]
          tunnel: "Stored Locations Array" -> [_ w205]
          frame False {
          }
          frame True {
            n64 = case shown="\"Drive\", Default" w206 {
              tunnel: w210 -> [w219 w232 w241 w258]
              tunnel: [w223 w232 w244 w263] -> w208
              tunnel: w209 -> [w220 w235 _ _]
              tunnel: [w222 w234 w245 w264] -> w207
              tunnel: w211 -> [w221 w233 w246 w262]
              tunnel: w205 -> [w214 w230 w240 w257]
              frame "Drive", Default {
                n65 = Index Array(array=w214, index="Waypoint Location") -> (element=w217:T5)
                n66 = call "Initialize.vi"("Tolerance (m)"=w220, "Drive Location"=w217) -> ("Drive out"=w215:refnum<class "DriveTo.lvclass">)  [unwired: 8 in, 1 out]
                n67 = Flatten To String(anything=w215) -> (data string=w213:string)  [unwired: 3 in, 2 out]
                n68 = Bundle By Name(cluster=T44 {"OCU Command"=enum."Add Mission", "Data"=variant}, "Data"=w213) -> (w212:T44)
                n69 = call "Write.vi"("error in (no error)"=w219, "element"=w212, "NetworkStreamWriter in"=w221) -> ("error out"=w223:errorcluster, "NetworkStreamWriter out"=w222:refnum<class "NetworkStreamWriter.lvclass">)  [unwired: 6 in, 1 out]
              }
              frame "Round" {
                n70 = Index Array(array=w230, index="Buoy to Round") -> (element=w229:T5)
                n71 = call "Initialize.vi"("Tolerance (m)"=w235, "Round side?"="Buoy Side", "Buoy to Round"=w229) -> ("RoundBuoys out"=w224:refnum<class "RoundBuoy.lvclass">)  [unwired: 7 in, 1 out]
                n72 = Flatten To String(anything=w224) -> (data string=w226:string)  [unwired: 3 in, 2 out]
                n73 = Bundle By Name(cluster=T44 {"OCU Command"=enum."Add Mission", "Data"=variant}, "Data"=w226) -> (w225:T44)
                n74 = call "Write.vi"("element"=w225, "NetworkStreamWriter in"=w233) -> ("NetworkStreamWriter out"=w234:refnum<class "NetworkStreamWriter.lvclass">)  [unwired: 7 in, 2 out]
              }
              frame "Pass" {
                # "build Pass Between Buoys mission"
                n75 = Index Array(array=w240, index #1="Starboard Buoy", index #2="Port Buoy") -> (element #1=w239:T5, element #2=w238:T5)
                n76 = call "Initialize.vi"("Buoy Pass 2"=w238, "Buoy Pass 1"=w239) -> ("PassBuoys out"=w242:refnum<class "PassBuoys.lvclass">)  [unwired: 8 in, 1 out]
                n77 = Flatten To String(anything=w242) -> (data string=w248:string)  [unwired: 3 in, 2 out]
                n78 = To Variant(anything=w248) -> (Variant=w249:variant)
                n79 = Bundle By Name(cluster=T44 {"OCU Command"=enum."Add Mission", "Data"=variant}, "Data"=w249) -> (w247:T44)
                n80 = To Variant(anything=w247) -> (Variant=w243:variant)
                n81 = call "Write.vi"("error in (no error)"=w241, "element"=w243, "NetworkStreamWriter in"=w246) -> ("error out"=w244:errorcluster, "NetworkStreamWriter out"=w245:refnum<class "NetworkStreamWriter.lvclass">)  [unwired: 6 in, 1 out]
              }
              frame "Station" {
                # "user inputs two points as a line and we convert it to a square"
                n82 = Index Array(array=w257, index #1="Buoy A", index #2="Buoy B") -> (element #1=w254:T5, element #2=w253:T5)
                n83 = call "helper - UTM line to Square.vi"("Endpoint 2, UTM"=w253, "Endpoint 1, UTM"=w254) -> ("Endpoint 4, UTM"=w260:T5, "Endpoint 3, UTM"=w259:T5)
                n84 = call "Initialize.vi"("Buoy SE"=w253, "Buoy SW"=w254, "Buoy NE"=w260, "Buoy NW"=w259) -> ("StationKeeping out"=w261:refnum<class "StationKeeping.lvclass">)  [unwired: 6 in, 1 out]
                n85 = Flatten To String(anything=w261) -> (data string=w252:string)  [unwired: 3 in, 2 out]
                n86 = Bundle By Name(cluster=T44 {"OCU Command"=enum."Add Mission", "Data"=variant}, "Data"=w252) -> (w251:T44)
                n87 = call "Write.vi"("error in (no error)"=w258, "element"=w251, "NetworkStreamWriter in"=w262) -> ("error out"=w263:errorcluster, "NetworkStreamWriter out"=w264:refnum<class "NetworkStreamWriter.lvclass">)  [unwired: 6 in, 1 out]
              }
            }
          }
        }
      }
      event "Boat to Point 0", "Boat to Point 1", "Boat to Point 2", "Boat to Point 3", "Boat to Point 4", "Local to Point 3", "Local to Point 2", "Local to Point 1", "Local to Point 0", "Local to Point 4": Value Change {
        # "save the current GPS location to one of the saved points."
        n88 = event-data() -> ()  [unwired: 1 in, 1 out]
        n89 = Build Array("Boat to Point 0", "Boat to Point 1", "Boat to Point 2", "Boat to Point 3", "Boat to Point 4") -> (w275:bool[])
        n90 = Build Array("Local to Point 0", "Local to Point 1", "Local to Point 2", "Local to Point 3", "Local to Point 4") -> (w266:bool[])
        n91 = for {
          tunnel: w275 -> [w288] mode=indexing
          i -> [w287]
          n92 = case shown="True" w288 {
            tunnel: w287 -> [_ w290]
            frame False {
            }
            frame True {
              # "load from boat GPS"
              n93 = local read "Stored Locations Array"() -> (w292:T5[])
              n94 = local read "Robot UTM Location"() -> (w289:T5)
              n95 = Replace Array Subset(array=w292, new element=w289, index=w290) -> (w291:T5[])
              n96 = local write "Stored Locations Array"(w291) -> ()
            }
          }
        }
        n97 = for {
          tunnel: w266 -> [w282] mode=indexing
          i -> [w281]
          n98 = case shown="True" w282 {
            tunnel: w281 -> [_ w283]
            frame False {
            }
            frame True {
              # "load from local GPS"
              n99 = local read "Stored Locations Array"() -> (w285:T5[])
              n100 = global read "2 Global.vi" "Robot UTM Location"() -> (w284:T5)
              n101 = Replace Array Subset(array=w285, new element=w284, index=w283) -> (w286:T5[])
              n102 = local write "Stored Locations Array"(w286) -> ()
            }
          }
        }
      }
      event "Update Constants": Value Change {
        # "To add a set of tuning constants, add a control constant in the cluster constant\nadd the control to the front panel and wire it into the bundler in the true case here; the  0x2 command\nreceive block will need to be edited as well as the TuningConstants global"
        n103 = event-data() -> ()  [unwired: 1 in, 1 out]
        n104 = case shown="True" "Update Constants" {
          tunnel: w296 -> [w300 w317]
          tunnel: w295 -> [w299 w316]
          tunnel: [w300 w315] -> w294
          tunnel: [w299 w314] -> w293
          frame False {
          }
          frame True {
            n105 = Bundle By Name(cluster=T46 {"Goodness Weightings"={"Target Importance"=0.0, "No Sail Importance"=0.0, "Change Importance"=0.0, "Pure Waypoint \nImportance"=0.0, "Pure Wind \nImportance"=0.0}, "PI Constants"={"Proportional Gain"=0.0, "Integral Time"=0.0, "Derivative Time"=0.0}, "No Sail Zone\nTuning Quotient"=0.0, "Heading Change Wind Adjustment"=0.0, "Waypoint Tuning Quotient"=0.0, "Apparent Wind Mode"={"Desired Apparent\nWind Direction"=0.0, "On"=FALSE}, "RP Autonomous"=FALSE, "Let Sail Out on Windcross"=FALSE, "Shift Goal for currents"=FALSE, "Round Buoy Safety"=0.0}, "Round Buoy Safety"="Round Buoy Safety", "RP Autonomous"="Runprotection Enabled", "Goodness Weightings"="Goodness Weightings", "PI Constants"="PI Constants", "No Sail Zone\nTuning Quotient"="No Sail Zone\nTuning Quotient", "Heading Change Wind Adjustment"="Heading Change\nWind Adjustment", "Waypoint Tuning Quotient"="Waypoint\nTuning Quotient", "Apparent Wind Mode"="Apparent Wind Mode", "Let Sail Out on Windcross"="Let Sail Out on Windcross", "Shift Goal for currents"="Shift Goal for currents") -> (w302:T46)
            n106 = Bundle By Name(cluster=T44 {"OCU Command"=enum."Edit Control Values", "Data"=variant}, "Data"=w302) -> (w301:T44)
            n107 = call "Write.vi"("error in (no error)"=w316, "element"=w301, "NetworkStreamWriter in"=w317) -> ("error out"=w314:errorcluster, "NetworkStreamWriter out"=w315:refnum<class "NetworkStreamWriter.lvclass">)  [unwired: 6 in, 1 out]
          }
        }
      }
      event "Log message": Key Up {
        # "Remove carriage\nreturn."
        # "Enter key?"
        n108 = event-data() -> ("ScanCode"=w320:i16)  [unwired: 1 in, 2 out]
        n109 = Equal?(x=w320, y=i16 28) -> (x = y?=w329:bool)
        n110 = Search and Replace String(replace all?=TRUE ("replace all? (F)"), input string="Log message", search string="\n" ("string"), replace string="") -> (result string=w326:string)  [unwired: 4 in, 3 out]
        n111 = case "Was the log message entered?" shown="True" w329 {
          tunnel: [w333 w342] -> w324
          tunnel: [w332 w341] -> w321
          tunnel: w323 -> [w332 w336]
          tunnel: w322 -> [w333 w340]
          tunnel: w326 -> [_ w337]
          frame False {
          }
          frame True {
            n112 = To Variant(anything=w337) -> (Variant=w344:variant)
            n113 = property on="Log message" class="Str"(error in=w336, "Value"="") -> (error out=w335:errorcluster)  [unwired: 1 in, 1 out]
            n114 = Bundle By Name(cluster=T44 {"OCU Command"=enum."Log Message", "Data"=variant}, "Data"=w344) -> (w343:T44)
            n115 = To Variant(anything=w343) -> (Variant=w338:variant)
            n116 = call "Write.vi"("error in (no error)"=w335, "element"=w338, "NetworkStreamWriter in"=w340) -> ("error out"=w341:errorcluster, "NetworkStreamWriter out"=w342:refnum<class "NetworkStreamWriter.lvclass">)  [unwired: 6 in, 1 out]
          }
        }
      }
      event "Save Waypoints\nand PoI": Value Change {
        n117 = event-data() -> ()  [unwired: 1 in, 1 out]
        n118 = case "Save MDF" shown="True" "Save Waypoints\nand PoI" {
          frame False {
          }
          frame True {
            n119 = local read "Global No Sail Circles"() -> (w349:T33[])
            n120 = local read "Mission Object Array"() -> (w350:refnum<class "GenericMission.lvclass">[])
            n121 = call "0-Write MDF.vi"("Global No Sail Circles"=w349, "Missions (Object Array)"=w350) -> ()  [unwired: 3 in, 1 out]
          }
        }
      }
      event "Load MDF": Value Change {
        n122 = event-data() -> ()  [unwired: 1 in, 1 out]
        n123 = case "Load MDF" shown="True" "Load MDF" {
          tunnel: w354 -> [w357 w360]
          tunnel: [w357 w367] -> w353
          tunnel: w352 -> [w358 w362]
          tunnel: [w358 w365] -> w351
          frame False {
          }
          frame True {
            w364 = T44 {"OCU Command"=enum."Reset Missions/Waypts", "Data"=variant}  # clear missions
            n124 = To Variant(anything=w364) -> (Variant=w363:variant)
            n125 = call "Write.vi"("error in (no error)"=w360, "element"=w363, "NetworkStreamWriter in"=w362) -> ("error out"=w359:errorcluster, "NetworkStreamWriter out"=w361:refnum<class "NetworkStreamWriter.lvclass">)  [unwired: 6 in, 1 out]
            n126 = call "0-Read MDF.vi"("Error in"=w359, "MDF file path"="Mission Def Filepath") -> ("Error out"=w369:errorcluster, "Global No Sail Circles"=w371:T33[], "Missions (Object Array)"=w370:refnum<class "GenericMission.lvclass">[])  [unwired: 1 in]
            n127 = for {
              tunnel: w370 -> [w382] mode=indexing
              shift-right: [w388] -> w368
              shift-left: w369 -> [w384]
              tunnel: w361 -> [w387]
              tunnel: [w386] -> w366
              n128 = Flatten To String(anything=w382, error in (no error)=w384) -> (data string=w383:string, error out=w385:errorcluster)  [unwired: 2 in, 1 out]
              n129 = To Variant(anything=w383) -> (Variant=w390:variant)
              n130 = Bundle By Name(cluster=T44 {"OCU Command"=enum."Add Mission", "Data"=variant}, "Data"=w390) -> (w391:T44)
              n131 = To Variant(anything=w391) -> (Variant=w389:variant)
              n132 = call "Write.vi"("error in (no error)"=w385, "element"=w389, "NetworkStreamWriter in"=w387) -> ("error out"=w388:errorcluster, "NetworkStreamWriter out"=w386:refnum<class "NetworkStreamWriter.lvclass">)  [unwired: 6 in, 1 out]
            }
            n133 = local write "Mission Object Array"(w370) -> ()
            n134 = local write "Global No Sail Circles"(w371) -> ()
            n135 = for {
              tunnel: w371 -> [w374] mode=indexing
              tunnel: w366 -> [w376]
              shift-right: [w377] -> w367
              shift-left: w368 -> [w373]
              tunnel: [w375] -> w365
              n136 = To Variant(anything=w374) -> (Variant=w379:variant)
              n137 = Bundle By Name(cluster=T44 {"OCU Command"=enum."Add Global No-Sail", "Data"=variant}, "Data"=w379) -> (w380:T44)
              n138 = To Variant(anything=w380) -> (Variant=w378:variant)
              n139 = call "Write.vi"("error in (no error)"=w373, "element"=w378, "NetworkStreamWriter in"=w376) -> ("error out"=w377:errorcluster, "NetworkStreamWriter out"=w375:refnum<class "NetworkStreamWriter.lvclass">)  [unwired: 6 in, 1 out]
            }
          }
        }
      }
      event "Reset Missions/Waypts": Value Change {
        n140 = event-data() -> ()  [unwired: 1 in, 1 out]
        n141 = case "Reset Missions" shown="True" "Reset Missions/Waypts" {
          tunnel: w396 -> [w400 w406]
          tunnel: w395 -> [w399 w405]
          tunnel: [w400 w404] -> w394
          tunnel: [w399 w403] -> w393
          frame False {
          }
          frame True {
            n142 = To Variant(anything=T44 {"OCU Command"=enum."Reset Missions/Waypts", "Data"=variant}) -> (Variant=w401:variant)
            n143 = call "Write.vi"("error in (no error)"=w405, "element"=w401, "NetworkStreamWriter in"=w406) -> ("error out"=w403:errorcluster, "NetworkStreamWriter out"=w404:refnum<class "NetworkStreamWriter.lvclass">)  [unwired: 6 in, 1 out]
          }
        }
      }
      event "Mission Map": Mouse Up {
        # "add a waypoint to the list"
        n144 = event-data() -> ()  [unwired: 1 in, 1 out]
        n145 = case shown="\"Go to Waypoint\", Default" w409 {
          selector: w409 -> [_ _ w489 _ _]
          tunnel: w414 -> [w425 w451 w496 w514 w534]
          tunnel: [w423 w461 w493 w505 w525] -> w412
          tunnel: w413 -> [w424 w448 w478 w500 w532]
          tunnel: w408 -> [w418 _ w490 _ w515]
          tunnel: [w421 w459 w482 w508 w526] -> w411
          tunnel: w410 -> [w420 w458 w479 w509 w524]
          tunnel: "Time(s)" -> [_ _ _ _ w516]
          frame "Go to Waypoint", Default {
            n146 = property on="Mission Map" class="ImageControl"(error in=w425) -> (error out=w427:errorcluster, "Last Mouse Position"=w426:cluster{"X":i32, "Y":i32})  [unwired: 1 in, 1 out]
            n147 = call "Helper - Image To UTM.vi"("Image Descriptor"=w424, "Pixel Coordinates"=w426) -> ("UTM Location"=w416:T5)  [unwired: 1 in, 1 out]
            n148 = invoke on="Mission Map" class="ImageControl" method="Clear ROI"(error in=w427) -> (error out=w422:errorcluster)  [unwired: 2 in, 2 out]
            n149 = disable-structure shown="Enabled" {
              disable-tunnel: w418 -> [w434 w437]
              disable-tunnel: [w430 w441] -> w417
              disable-tunnel: w416 -> [w428 w436]
              frame Enabled {
                n150 = call "Initialize.vi"("Tolerance (m)"=w434, "Drive Location"=w428) -> ("Drive out"=w429:refnum<class "DriveTo.lvclass">)  [unwired: 8 in, 1 out]
                n151 = Flatten To String(anything=w429) -> (data string=w431:string)  [unwired: 3 in, 2 out]
                n152 = To Variant(anything=w431) -> (Variant=w432:variant)
                n153 = Bundle By Name(cluster=T44 {"OCU Command"=enum."Add Mission", "Data"=variant}, "Data"=w432) -> (w430:T44)
              }
              frame Disabled {
                n154 = call "init_waypoint.vi"("Coords"=w436, "Tolerance (m)"=w437) -> ("Waypoint Out"=w435:refnum<class "Waypoint.lvclass">)  [unwired: 9 in]
                n155 = Flatten To String(anything=w435) -> (data string=w438:string)  [unwired: 3 in, 2 out]
                n156 = To Variant(anything=w438) -> (Variant=w439:variant)
                n157 = Bundle By Name(cluster=T44 {"OCU Command"=enum."Add waypoint", "Data"=variant}, "Data"=w439) -> (w441:T44)
              }
            }
            n158 = To Variant(anything=w417) -> (Variant=w419:variant)
            n159 = call "Write.vi"("error in (no error)"=w422, "element"=w419, "NetworkStreamWriter in"=w420) -> ("error out"=w423:errorcluster, "NetworkStreamWriter out"=w421:refnum<class "NetworkStreamWriter.lvclass">)  [unwired: 6 in, 1 out]
          }
          frame "Global No-Sail Zone" {
            n160 = property on="Mission Map" class="ImageControl"(error in=w451) -> (error out=w450:errorcluster, "ROI"=w452:T49)  [unwired: 1 in, 1 out]
            n161 = call "helper- line ROI to 2 UTM Pts.vi"("ROI"=w452, "Image Descriptor"=w448) -> ("Endpoint UTM 2"=w447:T5, "Endpoint UTM 1"=w449:T5)
            n162 = Unbundle By Name(w447) -> ("East"=w445:dbl, "North"=w446:dbl)
            n163 = Unbundle By Name(w449) -> ("UTM Zone"=w453:dbl, "Hemisphere"=w454:enum16{"North", "South"}, "East"=w443:dbl, "North"=w444:dbl)
            n164 = call "Helper - Distance Between Two Points.vi"("y 2"=w446, "x 2"=w445, "y"=w444, "x"=w443) -> ("Numeric"=w442:dbl)
            n165 = invoke on="Mission Map" class="ImageControl" method="Clear ROI"(error in=w450) -> (error out=w460:errorcluster)  [unwired: 2 in, 2 out]
            n166 = disable-structure shown="Enabled" {
              disable-tunnel: w442 -> [w467 w473]
              disable-tunnel: [w469 w477] -> w456
              disable-tunnel: T33 {"UTM Zone"=0.0, "Hemisphere"=enum."North", "East"=0.0, "North"=0.0, "Radius"=0.0} ("UTM Location") -> [w468 _]
              disable-tunnel: w444 -> [w466 _]
              disable-tunnel: w443 -> [w465 _]
              disable-tunnel: w454 -> [w464 _]
              disable-tunnel: w453 -> [w463 _]
              frame Enabled {
                n167 = Bundle By Name(cluster=w468, "UTM Zone"=w463, "Hemisphere"=w464, "East"=w465, "North"=w466, "Radius"=w467) -> (w462:T33)
                n168 = To Variant(anything=w462) -> (Variant=w470:variant)
                n169 = Bundle By Name(cluster=T44 {"OCU Command"=enum."Add Global No-Sail", "Data"=variant}, "Data"=w470) -> (w469:T44)
              }
              frame Disabled {
                n170 = call "init_waypoint.vi"("Tolerance (m)"=w473) -> ("Waypoint Out"=w472:refnum<class "Waypoint.lvclass">)  [unwired: 10 in]
                n171 = Flatten To String(anything=w472) -> (data string=w474:string)  [unwired: 3 in, 2 out]
                n172 = To Variant(anything=w474) -> (Variant=w475:variant)
                n173 = Bundle By Name(cluster=T44 {"OCU Command"=enum."Add waypoint", "Data"=variant}, "Data"=w475) -> (w477:T44)
              }
            }
            n174 = To Variant(anything=w456) -> (Variant=w457:variant)
            n175 = call "Write.vi"("error in (no error)"=w460, "element"=w457, "NetworkStreamWriter in"=w458) -> ("error out"=w461:errorcluster, "NetworkStreamWriter out"=w459:refnum<class "NetworkStreamWriter.lvclass">)  [unwired: 6 in, 1 out]
          }
          frame "Round Buoy Starboard", "Round Buoy Port" {
            n176 = property on="Mission Map" class="ImageControl"(error in=w496) -> (error out=w498:errorcluster, "Last Mouse Position"=w497:cluster{"X":i32, "Y":i32})  [unwired: 1 in, 1 out]
            n177 = Equal?(x=w489, y=Mission_Type_Radio_Buttons."Round Buoy Port" ("Mission Type 2")) -> (x = y?=w484:bool)
            n178 = call "Helper - Image To UTM.vi"("Image Descriptor"=w478, "Pixel Coordinates"=w497) -> ("UTM Location"=w491:T5)  [unwired: 1 in, 1 out]
            n179 = invoke on="Mission Map" class="ImageControl" method="Clear ROI"(error in=w498) -> (error out=w493:errorcluster)  [unwired: 2 in, 2 out]
            n180 = Select(t=enum16{"Starboard", "Port"}."Port" ("Round side?"), s=w484, f=enum16{"Starboard", "Port"}."Starboard" ("Round side?")) -> (s? t:f=w485:enum16{"Starboard", "Port"})
            n181 = call "Initialize.vi"("Tolerance (m)"=w490, "Round side?"=w485, "Buoy to Round"=w491) -> ("RoundBuoys out"=w483:refnum<class "RoundBuoy.lvclass">)  [unwired: 7 in, 1 out]
            n182 = Flatten To String(anything=w483) -> (data string=w492:string)  [unwired: 3 in, 2 out]
            n183 = To Variant(anything=w492) -> (Variant=w494:variant)
            n184 = Bundle By Name(cluster=T44 {"OCU Command"=enum."Add Mission", "Data"=variant}, "Data"=w494) -> (w480:T44)
            n185 = To Variant(anything=w480) -> (Variant=w481:variant)
            n186 = call "Write.vi"("element"=w481, "NetworkStreamWriter in"=w479) -> ("NetworkStreamWriter out"=w482:refnum<class "NetworkStreamWriter.lvclass">)  [unwired: 7 in, 2 out]
          }
          frame "Pass Between Buoys" {
            # "build Pass Between Buoys mission"
            n187 = property on="Mission Map" class="ImageControl"(error in=w514) -> (error out=w506:errorcluster, "ROI"=w499:T49)  [unwired: 1 in, 1 out]
            n188 = invoke on="Mission Map" class="ImageControl" method="Clear ROI"(error in=w506) -> (error out=w507:errorcluster)  [unwired: 2 in, 2 out]
            n189 = call "helper- line ROI to 2 UTM Pts.vi"("ROI"=w499, "Image Descriptor"=w500) -> ("Endpoint UTM 2"=w502:T5, "Endpoint UTM 1"=w501:T5)
            n190 = call "Initialize.vi"("Buoy Pass 2"=w502, "Buoy Pass 1"=w501) -> ("PassBuoys out"=w503:refnum<class "PassBuoys.lvclass">)  [unwired: 8 in, 1 out]
            n191 = Flatten To String(anything=w503) -> (data string=w511:string)  [unwired: 3 in, 2 out]
            n192 = To Variant(anything=w511) -> (Variant=w512:variant)
            n193 = Bundle By Name(cluster=T44 {"OCU Command"=enum."Add Mission", "Data"=variant}, "Data"=w512) -> (w510:T44)
            n194 = To Variant(anything=w510) -> (Variant=w504:variant)
            n195 = call "Write.vi"("error in (no error)"=w507, "element"=w504, "NetworkStreamWriter in"=w509) -> ("error out"=w505:errorcluster, "NetworkStreamWriter out"=w508:refnum<class "NetworkStreamWriter.lvclass">)  [unwired: 6 in, 1 out]
          }
          frame "Station Keeping" {
            # "user inputs two points as a line and we convert it to a square"
            n196 = property on="Mission Map" class="ImageControl"(error in=w534) -> (error out=w522:errorcluster, "ROI"=w533:T49)  [unwired: 1 in, 1 out]
            n197 = call "helper- line ROI to 2 UTM Pts.vi"("ROI"=w533, "Image Descriptor"=w532) -> ("Endpoint UTM 2"=w517:T5, "Endpoint UTM 1"=w518:T5)
            n198 = call "helper - UTM line to Square.vi"("Endpoint 2, UTM"=w517, "Endpoint 1, UTM"=w518) -> ("Endpoint 4, UTM"=w520:T5, "Endpoint 3, UTM"=w519:T5)
            n199 = invoke on="Mission Map" class="ImageControl" method="Clear ROI"(error in=w522) -> (error out=w523:errorcluster)  [unwired: 2 in, 2 out]
            n200 = call "Initialize.vi"("Tolerance (m)"=w515, "Duration (s)"=w516, "Buoy SE"=w517, "Buoy SW"=w518, "Buoy NE"=w520, "Buoy NW"=w519) -> ("StationKeeping out"=w521:refnum<class "StationKeeping.lvclass">)  [unwired: 4 in, 1 out]
            n201 = Flatten To String(anything=w521) -> (data string=w529:string)  [unwired: 3 in, 2 out]
            n202 = To Variant(anything=w529) -> (Variant=w530:variant)
            n203 = Bundle By Name(cluster=T44 {"OCU Command"=enum."Add Mission", "Data"=variant}, "Data"=w530) -> (w528:T44)
            n204 = To Variant(anything=w528) -> (Variant=w527:variant)
            n205 = call "Write.vi"("error in (no error)"=w523, "element"=w527, "NetworkStreamWriter in"=w524) -> ("error out"=w525:errorcluster, "NetworkStreamWriter out"=w526:refnum<class "NetworkStreamWriter.lvclass">)  [unwired: 6 in, 1 out]
          }
        }
      }
      event Value Change {
        # "gray out the appropriate numeric controls"
        # "set input tool"
        # "Adjust OCU controls for the correct mission input style"
        n206 = event-data() -> ("NewVal"=w540:T14)  [unwired: 1 in]
        n207 = case shown="\"Station Keeping\"" w540 {
          tunnel: [T47."Enabled" ("Disabled") w544 T47."Enabled" ("Disabled")] -> w539
          tunnel: [T47."Disabled and Grayed Out" ("Disabled") w544 T47."Enabled" ("Disabled")] -> w538
          frame "Go to Waypoint", Default {
          }
          frame "Pass Between Buoys", "Global No-Sail Zone" {
            w544 = T47."Disabled and Grayed Out" ("Disabled")
            # "\"Pass Between Buoys\"\nhas neither input"
          }
          frame "Station Keeping" {
          }
        }
        n208 = case shown="\"Pass Between Buoys\", \"Global No-Sail Zone\"" w540 {
          tunnel: [w547 w548 w549] -> w541
          frame "Go to Waypoint", Default {
            w547 = u32 1 items=["Zoom Tool"=8, "Selection Tool"=0, "Pan Tool"=9, "Point Tool"=1, "Line Tool"=2, "Rectangle Tool"=3, "Rotated Rectangle Tool"=12, "Polyline Tool"=10, "Polygon Tool"=5, "Freehand Tool"=11, "Closed Freehand Tool"=6, "Ellipse Tool"=4, "Annulus Tool"=7] ("Current ROI Tool")
          }
          frame "Station Keeping" {
            w548 = u32 2 items=["Zoom Tool"=8, "Selection Tool"=0, "Pan Tool"=9, "Point Tool"=1, "Line Tool"=2, "Rectangle Tool"=3, "Rotated Rectangle Tool"=12, "Polyline Tool"=10, "Polygon Tool"=5, "Freehand Tool"=11, "Closed Freehand Tool"=6, "Ellipse Tool"=4, "Annulus Tool"=7] ("Current ROI Tool")
          }
          frame "Pass Between Buoys", "Global No-Sail Zone" {
            w549 = u32 2 items=["Zoom Tool"=8, "Selection Tool"=0, "Pan Tool"=9, "Point Tool"=1, "Line Tool"=2, "Rectangle Tool"=3, "Rotated Rectangle Tool"=12, "Polyline Tool"=10, "Polygon Tool"=5, "Freehand Tool"=11, "Closed Freehand Tool"=6, "Ellipse Tool"=4, "Annulus Tool"=7] ("Current ROI Tool")
          }
        }
        n209 = property on="Tolerance" class="DigNum (strict)"("DisabledEnum"=w539) -> ()  [unwired: 2 in, 2 out]
        n210 = property on="Time(s)" class="DigNum (strict)"("DisabledEnum"=w538) -> ()  [unwired: 2 in, 2 out]
        n211 = property on="Mission Map" class="ImageControl"("Current ROI Tool"=w541) -> ()  [unwired: 2 in, 2 out]
      }
    }
    n212 = local read "Setpoints to boat"() -> (w101:T26)
    n213 = local read "OVERRIDE RUDDER?"() -> (w107:bool)
    n214 = local read "OVERRIDE SAIL?"() -> (w102:bool)
    n215 = Unbundle By Name(w109) -> ("Sail Position"=w104:T27, "Rudder Angle"=w105:T28)
    n216 = Unbundle By Name(w101) -> ("Sail Position"=w100:T27, "Rudder Angle"=w99:T28)
    n217 = call "eStopShared.vi"("Command"=eStopCommand."Set E-Stop", "E-Stop"="Stop") -> ("E-Stop Out"=w114:bool)  [unwired: 8 in, 1 out]
    n218 = Select(t=w104, s=w102, f=w100) -> (s? t:f=→"Sail Position":T27)
    n219 = Select(t=w105, s=w107, f=w99) -> (s? t:f=→"Rudder Position":T28)
  }
  n220 = while {
    stop <- w559 stop-if-true
    n221 = global read "2 Global.vi" "Sensor Status"() -> (w557:T1)
    "Sensor Status" <- w557
    n222 = Unbundle By Name(w557) -> ("Sensor OK"=w553:T2, "Sensor Initialized"=w552:T2, "GPS Lock"=w550:T2)
    n223 = And(x=w553, y=w552) -> (x .and. y?=w551:T2)
    n224 = case shown="False" "Enable \nLocal GPS" {
      tunnel: w551 -> [_ w562]
      frame False {
        n225 = Wait Until Next ms Multiple(millisecond multiple=u32 100) -> ()  [unwired: 1 out]
      }
      frame True {
        n226 = case shown="False" w562 {
          tunnel: [w569 w571] -> w566
          tunnel: "GPS COM port" -> [w570 w571]
          tunnel: [w568 _] -> w564
          frame False {
            n227 = call "1A Helper - Init Sensor.vi"("VISA Refnum in"=w570) -> ("error out"=w568:errorcluster, "VISA Refnum out"=w569:refnum<visa-resource-name>)  [unwired: 8 in, 1 out]
          }
          frame True {
          }
        }
        n228 = call "1A Read Sensor Data.vi"("error (in)"=w564, "VISA resource name (in)"=w566) -> ("error (out)"=w563:errorcluster)  [unwired: 8 in, 1 out]
        n229 = case shown="Error" w563 {
          frame No Error {
          }
          frame Error {
            n230 = local write "Enable \nLocal GPS"(FALSE ("Enable \nLocal GPS")) -> ()
          }
        }
      }
    }
    n231 = call "eStopShared.vi"("Command"=eStopCommand."Get E-Stop") -> ("E-Stop Out"=w559:bool)  [unwired: 9 in, 1 out]
    n232 = Select(t=T47."Enabled" ("Disabled"), s=w550, f=T47."Disabled and Grayed Out" ("Disabled")) -> (s? t:f=w554:T47)
    n233 = property on="Local to Point 0" class="Bool"("DisabledEnum"=w554) -> ()  [unwired: 2 in, 2 out]
    n234 = property on="Local to Point 1" class="Bool"("DisabledEnum"=w554) -> ()  [unwired: 2 in, 2 out]
    n235 = property on="Local to Point 2" class="Bool"("DisabledEnum"=w554) -> ()  [unwired: 2 in, 2 out]
    n236 = property on="Local to Point 3" class="Bool"("DisabledEnum"=w554) -> ()  [unwired: 2 in, 2 out]
    n237 = property on="Local to Point 4" class="Bool"("DisabledEnum"=w554) -> ()  [unwired: 2 in, 2 out]
  }
  n238 = call "Close.vi"("error in (no error)"=w24, "NetworkStreamReader in"=w25) -> ()  [unwired: 8 in, 2 out]
  n239 = call "Close.vi"("error in (no error)"=w18, "NetworkStreamWriter in"=w19) -> ()  [unwired: 8 in, 2 out]
